vi "Generate Command Data Array.vi"(0 "Start Time (s)":dbl, 5 "End Time (s)":dbl) -> (4 "Array":string[](array[string]))   [LabVIEW 2025]
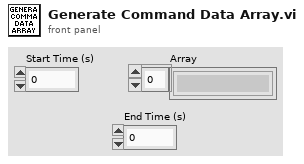
[diagram p1: front panel]
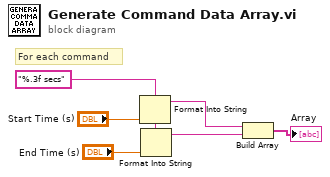
[diagram p0: block diagram]
diagram:
  w3 = "%.3f secs" ("format string")
  # "For each command"
  n1 = Format Into String(format string=w3, "Start Time (s)") -> (resulting string=w5:string)  [unwired: 2 in, 1 out]
  n2 = Format Into String(format string=w3, "End Time (s)") -> (resulting string=w1:string)  [unwired: 2 in, 1 out]
  n3 = Build Array(w5, w1) -> (→"Array":string[])
